vi "roboRIO v1.0 Config DI IRQ.vi"(5 "Enable IRQ?":bool, 6 "Edge Count":u32, 7 "IRQ Number":u8, 8 "error in (no error)":errorcluster, 9 "IO IRQ Channels Enum":T1, 10 "IRQ Type":T3, 11 "myRIO FPGA Ref In":T2) -> (0 "error out":errorcluster)   [LabVIEW 2021]
uses:
  <vilib>/myRIO/Common/Instrument Driver Framework/myRIO v1.0/IRQ/typedefs/IRQ Type.ctl
  <vilib>/myRIO/Common/Instrument Driver Framework/Utilities/typedefs/Generic FPGA Reference.ctl
  <vilib>/myRIO/Common/Instrument Driver Framework/myRIO v1.0/IRQ/typedefs/IO IRQ Channels Enum.ctl
  <vilib>/myRIO/Common/Instrument Driver Framework/roboRIO v1.0/IRQ/typedefs/roboRIO DI IRQ FPGA Reference.ctl
  <vilib>/Utility/error.llb/Error Cluster From Error Code.vi
  <vilib>/rvi/errors/niLvFpgaAdjustHostInterfaceError.vi
  <vilib>/rvi/interface/nirviReadWriteControl/nirviReadWriteControl.xnode
  <vilib>/rvi/interface/Simulation/niFpgaSimulationCallBeginRW.vi
  NiFpgaLv.dll
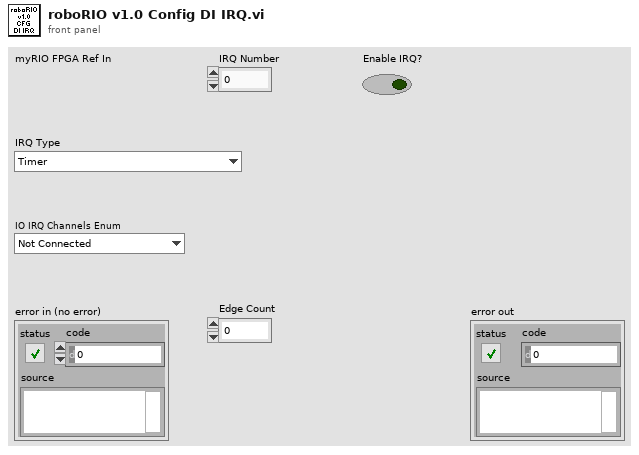
[diagram p1: front panel]
types:
  T1 = typedef "IO IRQ Channels Enum.ctl" = enum16{"Not Connected", "A/AI0 (Interrupt)", "A/AI1 (Interrupt)", "A/DIO0 (Interrupt)", "A/DIO1 (Interrupt)", "A/DIO2 (Interrupt)", "A/DIO3 (Interrupt)", "Button0 (Interrupt)", "B/AI0 (Interrupt)", "B/AI1 (Interrupt)", "B/DIO0 (Interrupt)", "B/DIO1 (Interrupt)", "B/DIO2 (Interrupt)", "B/DIO3 (Interrupt)"}
  T2 = typedef "Generic FPGA Reference.ctl" = refnum<k20>
  T3 = typedef "IRQ Type.ctl" = enum16{"Timer", "Analog falling edge", "Analog rising edge", "Digital falling edge", "Digital rising edge", "Digital edge"}
  T4 = typedef "roboRIO DI IRQ FPGA Reference.ctl" = refnum<k20>
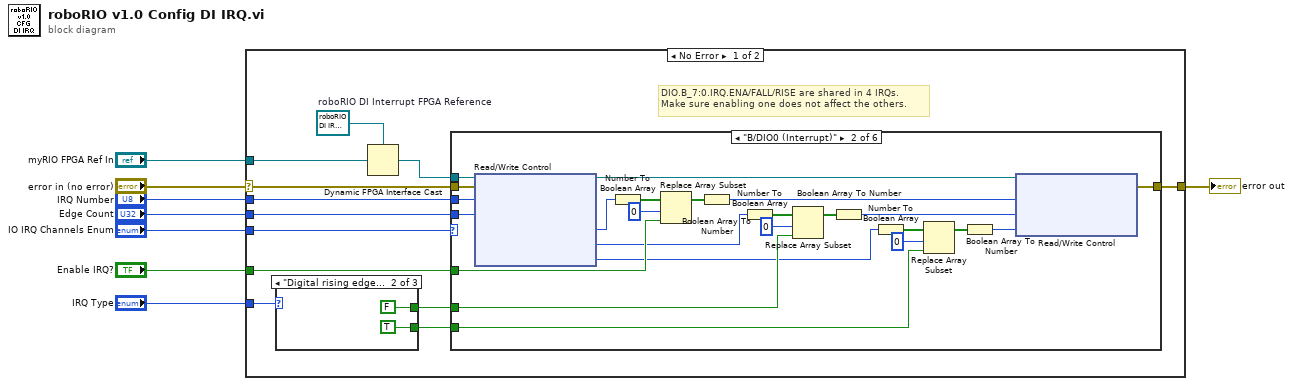
[diagram p0: block diagram]
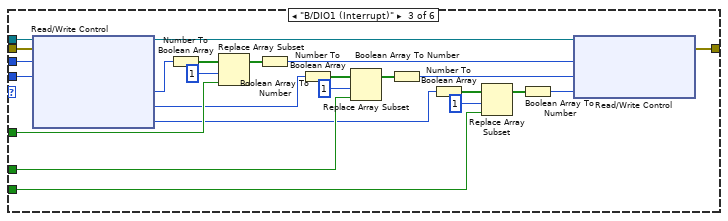
[diagram p3: hidden frame]
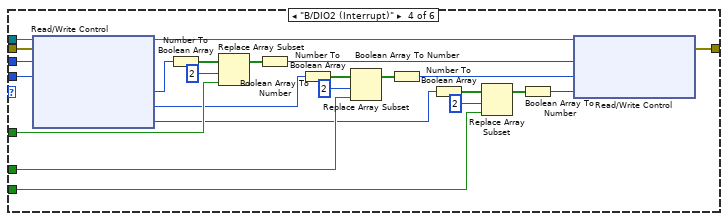
[diagram p4: hidden frame]
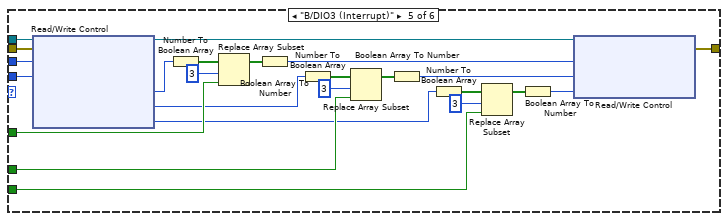
[diagram p5: hidden frame]
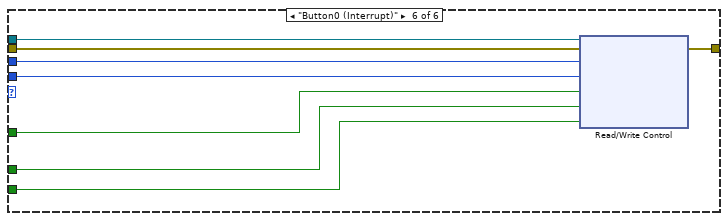
[diagram p6: hidden frame]
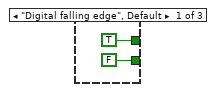
[diagram p7: hidden frame]
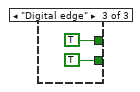
[diagram p8: hidden frame]
diagram:
  n1 = case shown="No Error" "error in (no error)" {
    selector: "error in (no error)" -> [w16 w132]
    tunnel: [w9 w132] -> w8
    tunnel: "IRQ Type" -> [w18 _]
    tunnel: "IRQ Number" -> [w15 _]
    tunnel: "myRIO FPGA Ref In" -> [w20 _]
    tunnel: "IO IRQ Channels Enum" -> [w13 _]
    tunnel: "Edge Count" -> [w14 _]
    tunnel: "Enable IRQ?" -> [w12 _]
    frame No Error {
      w19 = T4 refnum  # roboRIO DI Interrupt FPGA Reference
      # "DIO.B_7:0.IRQ.ENA/FALL/RISE are shared in 4 IRQs.\nMake sure enabling one does not affect the others."
      n2 = case shown="\"Digital rising edge\"" w18 {
        tunnel: [TRUE FALSE TRUE] -> w11
        tunnel: [FALSE TRUE TRUE] -> w10
        frame "Digital falling edge", Default {
        }
        frame "Digital rising edge" {
        }
        frame "Digital edge" {
        }
      }
      n3 = Dynamic FPGA Interface Cast(Session In=w19, Type=w20) -> (Session Out=w17:T4)
      n4 = case shown="\"B/DIO0 (Interrupt)\"" w13 {
        tunnel: w17 -> [_ w29 w53 w81 w105 w125]
        tunnel: w15 -> [_ w27 w51 w79 w103 w123]
        tunnel: w14 -> [_ w26 w50 w78 w102 w122]
        tunnel: w16 -> [w21 w28 w52 w80 w104 w124]
        tunnel: [w21 w30 w54 w74 w98 w118] -> w9
        tunnel: w11 -> [_ w35 w59 w83 w107 w120]
        tunnel: w10 -> [_ w34 w58 w82 w106 w119]
        tunnel: w12 -> [_ w42 w66 w90 w114 w121]
        frame Default {
        }
        frame "B/DIO0 (Interrupt)" {
          n5 = xnode "Read/Write Control"("FPGA VI Reference In"=w29, "error in"=w28, "IRQ.DIO_B_0.NO"=w27, "IRQ.DIO_B_0.CNT"=w26) -> ("FPGA VI Reference Out"=w25:T4, "IRQ.DIO_B_7:0.ENA"=w24:u8, "IRQ.DIO_B_7:0.FALL"=w23:u8, "IRQ.DIO_B_7:0.RISE"=w22:u8)  [unwired: 1 out]
          n6 = Number To Boolean Array(number=w24) -> (Boolean array=w44:bool[])
          n7 = Replace Array Subset(array=w44, new element=w42, index=0) -> (w45:bool[])
          n8 = Boolean Array To Number(Boolean array=w45) -> (number=w33:u8)
          n9 = Number To Boolean Array(number=w23) -> (Boolean array=w40:bool[])
          n10 = Replace Array Subset(array=w40, new element=w35, index=0) -> (w39:bool[])
          n11 = Boolean Array To Number(Boolean array=w39) -> (number=w32:u8)
          n12 = Number To Boolean Array(number=w22) -> (Boolean array=w37:bool[])
          n13 = Replace Array Subset(array=w37, new element=w34, index=0) -> (w38:bool[])
          n14 = Boolean Array To Number(Boolean array=w38) -> (number=w31:u8)
          n15 = xnode "Read/Write Control"("FPGA VI Reference In"=w25, "IRQ.DIO_B_7:0.ENA"=w33, "IRQ.DIO_B_7:0.FALL"=w32, "IRQ.DIO_B_7:0.RISE"=w31) -> ("error out"=w30:errorcluster)  [unwired: 1 in, 1 out]
        }
        frame "B/DIO1 (Interrupt)" {
          n16 = xnode "Read/Write Control"("FPGA VI Reference In"=w53, "error in"=w52, "IRQ.DIO_B_1.NO"=w51, "IRQ.DIO_B_1.CNT"=w50) -> ("FPGA VI Reference Out"=w49:T4, "IRQ.DIO_B_7:0.ENA"=w48:u8, "IRQ.DIO_B_7:0.FALL"=w47:u8, "IRQ.DIO_B_7:0.RISE"=w46:u8)  [unwired: 1 out]
          n17 = Number To Boolean Array(number=w48) -> (Boolean array=w68:bool[])
          n18 = Replace Array Subset(array=w68, new element=w66, index=1) -> (w69:bool[])
          n19 = Boolean Array To Number(Boolean array=w69) -> (number=w57:u8)
          n20 = Number To Boolean Array(number=w47) -> (Boolean array=w64:bool[])
          n21 = Replace Array Subset(array=w64, new element=w59, index=1) -> (w63:bool[])
          n22 = Boolean Array To Number(Boolean array=w63) -> (number=w56:u8)
          n23 = Number To Boolean Array(number=w46) -> (Boolean array=w61:bool[])
          n24 = Replace Array Subset(array=w61, new element=w58, index=1) -> (w62:bool[])
          n25 = Boolean Array To Number(Boolean array=w62) -> (number=w55:u8)
          n26 = xnode "Read/Write Control"("FPGA VI Reference In"=w49, "IRQ.DIO_B_7:0.ENA"=w57, "IRQ.DIO_B_7:0.FALL"=w56, "IRQ.DIO_B_7:0.RISE"=w55) -> ("error out"=w54:errorcluster)  [unwired: 1 in, 1 out]
        }
        frame "B/DIO2 (Interrupt)" {
          n27 = xnode "Read/Write Control"("FPGA VI Reference In"=w81, "error in"=w80, "IRQ.DIO_B_2.NO"=w79, "IRQ.DIO_B_2.CNT"=w78) -> ("FPGA VI Reference Out"=w73:T4, "IRQ.DIO_B_7:0.ENA"=w77:u8, "IRQ.DIO_B_7:0.FALL"=w76:u8, "IRQ.DIO_B_7:0.RISE"=w75:u8)  [unwired: 1 out]
          n28 = Number To Boolean Array(number=w77) -> (Boolean array=w92:bool[])
          n29 = Replace Array Subset(array=w92, new element=w90, index=2) -> (w93:bool[])
          n30 = Boolean Array To Number(Boolean array=w93) -> (number=w72:u8)
          n31 = Number To Boolean Array(number=w76) -> (Boolean array=w88:bool[])
          n32 = Replace Array Subset(array=w88, new element=w83, index=2) -> (w87:bool[])
          n33 = Boolean Array To Number(Boolean array=w87) -> (number=w71:u8)
          n34 = Number To Boolean Array(number=w75) -> (Boolean array=w85:bool[])
          n35 = Replace Array Subset(array=w85, new element=w82, index=2) -> (w86:bool[])
          n36 = Boolean Array To Number(Boolean array=w86) -> (number=w70:u8)
          n37 = xnode "Read/Write Control"("FPGA VI Reference In"=w73, "IRQ.DIO_B_7:0.ENA"=w72, "IRQ.DIO_B_7:0.FALL"=w71, "IRQ.DIO_B_7:0.RISE"=w70) -> ("error out"=w74:errorcluster)  [unwired: 1 in, 1 out]
        }
        frame "B/DIO3 (Interrupt)" {
          n38 = xnode "Read/Write Control"("FPGA VI Reference In"=w105, "error in"=w104, "IRQ.DIO_B_3.NO"=w103, "IRQ.DIO_B_3.CNT"=w102) -> ("FPGA VI Reference Out"=w97:T4, "IRQ.DIO_B_7:0.ENA"=w101:u8, "IRQ.DIO_B_7:0.FALL"=w100:u8, "IRQ.DIO_B_7:0.RISE"=w99:u8)  [unwired: 1 out]
          n39 = Number To Boolean Array(number=w101) -> (Boolean array=w116:bool[])
          n40 = Replace Array Subset(array=w116, new element=w114, index=3) -> (w117:bool[])
          n41 = Boolean Array To Number(Boolean array=w117) -> (number=w96:u8)
          n42 = Number To Boolean Array(number=w100) -> (Boolean array=w112:bool[])
          n43 = Replace Array Subset(array=w112, new element=w107, index=3) -> (w111:bool[])
          n44 = Boolean Array To Number(Boolean array=w111) -> (number=w95:u8)
          n45 = Number To Boolean Array(number=w99) -> (Boolean array=w109:bool[])
          n46 = Replace Array Subset(array=w109, new element=w106, index=3) -> (w110:bool[])
          n47 = Boolean Array To Number(Boolean array=w110) -> (number=w94:u8)
          n48 = xnode "Read/Write Control"("FPGA VI Reference In"=w97, "IRQ.DIO_B_7:0.ENA"=w96, "IRQ.DIO_B_7:0.FALL"=w95, "IRQ.DIO_B_7:0.RISE"=w94) -> ("error out"=w98:errorcluster)  [unwired: 1 in, 1 out]
        }
        frame "Button0 (Interrupt)" {
          n49 = xnode "Read/Write Control"("FPGA VI Reference In"=w125, "error in"=w124, "IRQ.DI_BTN.NO"=w123, "IRQ.DI_BTN.CNT"=w122, "IRQ.DI_BTN.ENA"=w121, "IRQ.DI_BTN.FALL"=w120, "IRQ.DI_BTN.RISE"=w119) -> ("error out"=w118:errorcluster)  [unwired: 1 out]
        }
      }
    }
    frame Error {
    }
  }
  "error out" <- w8
